vi "Divider3.vi"() -> (8 "Divider3":refnum<class "Divider3.lvclass">)   [LabVIEW 2017, in "Divider3.lvclass"]
uses:
  Divider3.lvclass
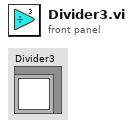
[diagram p1: front panel]
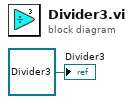
[diagram p0: block diagram]
diagram:
  "Divider3" <- refnum<class "Divider3.lvclass"> refnum ("Divider3.lvclass")
